vi "Untitled 2.vi"() -> ()   [LabVIEW 2018]
panel:
  out "freq":dbl
  in  "des max":dbl format="%#_13g"
  in  "a max":dbl format="%#_13g"
  in  "distância":dbl format="%#_13g"
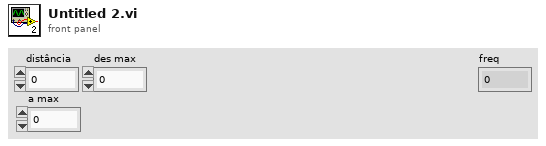
[diagram p1: front panel]
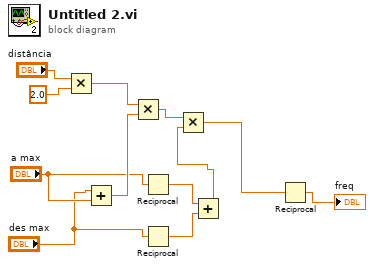
[diagram p0: block diagram]
diagram:
  n1 = Multiply(x="distância", y=2.0) -> (x*y=w10:dbl)
  n2 = Add(x="des max", y="a max") -> (x+y=w9:dbl)
  n3 = Multiply(x=w10, y=w9) -> (x*y=w8:dbl)
  n4 = Reciprocal(x="a max") -> (1/x=w5:dbl)
  n5 = Reciprocal(x="des max") -> (1/x=w4:dbl)
  n6 = Add(x=w5, y=w4) -> (x+y=w3:dbl)
  n7 = Multiply(x=w8, y=w3) -> (x*y=w2:dbl)
  n8 = Reciprocal(x=w2) -> (1/x=→"freq":dbl)
